vi "ElbowEncoderToAngle.vi"(0 "ElbowencoderPulses":i32, 1 "ShoulderAngle":dbl) -> (7 "elbow angle(deg)":dbl, 9 "Theta3":dbl)   [LabVIEW 2018]
uses:
  Arm Constants.vi
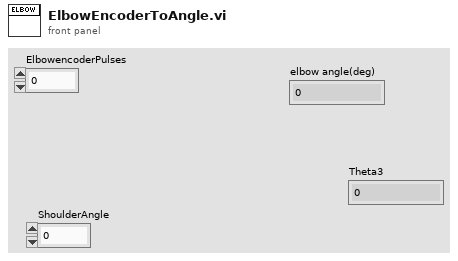
[diagram p1: front panel]
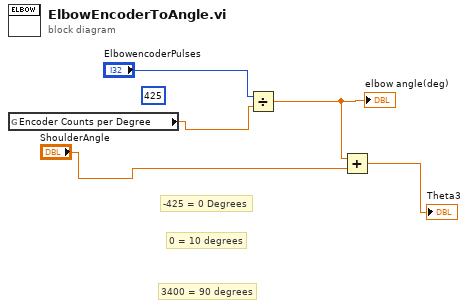
[diagram p0: block diagram]
diagram:
  (unwired) 425 ("y")
  # "-425 = 0 Degrees"
  # "0 = 10 degrees"
  # "3400 = 90 degrees"
  n1 = global read "Arm Constants.vi" "Encoder Counts per Degree"() -> (w1:dbl)
  n2 = Divide(x="ElbowencoderPulses", y=w1) -> (x/y=w4:dbl)
  "elbow angle(deg)" <- w4
  n3 = Add(x=w4, y="ShoulderAngle") -> (x+y=→"Theta3":dbl)
